vi "Periodic Tasks.vi"(8 "error in":errorcluster) -> ()   [LabVIEW 2012]
doc: "This VI runs in parallel to other tasks. It can contain as many user-defined periodic loops as you need. These can carry out PID or other sorts of timed response."
uses:
  <vilib>/Rock Robotics/SystemInterfaces/Utilities/FPGA_UtilitiesLED Source.ctl
  <vilib>/Rock Robotics/SystemInterfaces/Utilities/FPGA_UtilitiesLED State.ctl
  <vilib>/Rock Robotics/WPI/Compressor/WPI_CompressorGetSetRefNum.vi
  Robot Global Data.vi
panel:
  out "Shooter Speed":dbl
  out "Shooter Distance":dbl
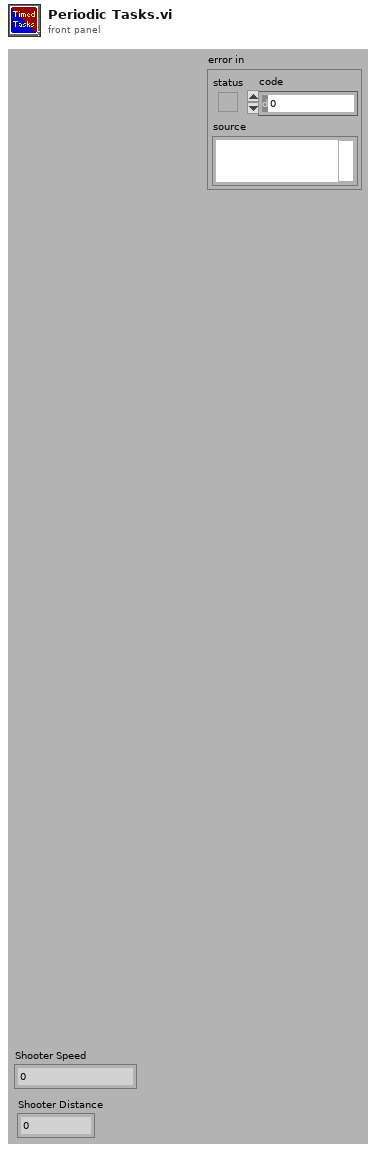
[diagram p1: front panel]
types:
  T1 = typedef "WPI_DriverStationRobotMode2.ctl" = enum16{"Autonomous Disabled", "Autonomous Enabled", "Teleop Disabled", "Teleop Enabled", "Timeout", "Finish", "Test Disabled", "Test Enabled"}
  T2 = typedef "WPI_EncoderDevRef.ctl" = cluster{"DevStatus":errorcluster, "EncoderIndex":T3, "CounterIndex":T4, "DistancePerCount":dbl, "Decoding Type":T5}
  T3 = typedef "FPGA_EncoderIdx.ctl" = enum8{"Enc 0", "Enc 1", "Enc 2", "Enc 3", "Invalid"}
  T4 = typedef "FPGA_CounterCtrSystemIndex.ctl" = enum8{"Ctr 0", "Ctr 1", "Ctr 2", "Ctr 3", "Ctr 4", "Ctr 5", "Ctr 6", "Ctr 7", "Invalid"}
  T5 = typedef "WPI_EncoderType.ctl" = enum16{"1x", "2x", "4x"}
  T6 = enum16{"Off", "Close Pyramid 3pt", "Far Pyramid 3pt", "Feeder Shot"}
  T7 = typedef "WPI_GyroDevRef.ctl" = cluster{"DevStatus":errorcluster, "Analog Module":T8, "Analog Channel":T9, "Offset":dbl, "Gain (VoltsPerDegree/Second)":dbl}
  T8 = typedef "FPGA_TypedefAnalogModule.ctl" = enum16{"Analog Module 1", "Analog Module 2"}
  T9 = typedef "FPGA_AIChannel.ctl" = enum8{"AI 1", "AI 2", "AI 3", "AI 4", "AI 5", "AI 6", "AI 7", "AI 8", "Invalid"}
  T10 = typedef "FPGA_UtilitiesLED State.ctl" = enum16{"Off", "On", "Toggle"}
  T11 = typedef "FPGA_UtilitiesLED Source.ctl" = enum16{"User LED", "FPGA LED"}
  T12 = typedef "WPI_CompressorDevRef.ctl" = cluster{"DevStatus":errorcluster, "DigitalInputDevRef":T13, "RelayDevRef":T16}
  T13 = typedef "WPI_DigitalInputDevRef.ctl" = cluster{"DevStatus":errorcluster, "DIO Channel":T14, "Digital Module":T15}
  T14 = typedef "FPGA_DIOChannel.ctl" = enum8{"DIO 1", "DIO 2", "DIO 3", "DIO 4", "DIO 5", "DIO 6", "DIO 7", "DIO 8", "DIO 9", "DIO 10", "DIO 11", "DIO 12", "DIO 13", "DIO 14", "Invalid"}
  T15 = typedef "FPGA_TypedefDigitalModule.ctl" = enum16{"Digital Module 1", "Digital Module 2"}
  T16 = typedef "WPI_RelayDevRef.ctl" = cluster{"DevStatus":errorcluster, "Relay Channel":T17, "Digital Module":T15, "Relay Direction":T18}
  T17 = typedef "FPGA_DIORelayChannel.ctl" = enum8{"Relay 1", "Relay 2", "Relay 3", "Relay 4", "Relay 5", "Relay 6", "Relay 7", "Relay 8", "Invalid"}
  T18 = typedef "WPI_RelayDirection.ctl" = enum16{"Both directions", "Forward only", "Reverse only"}
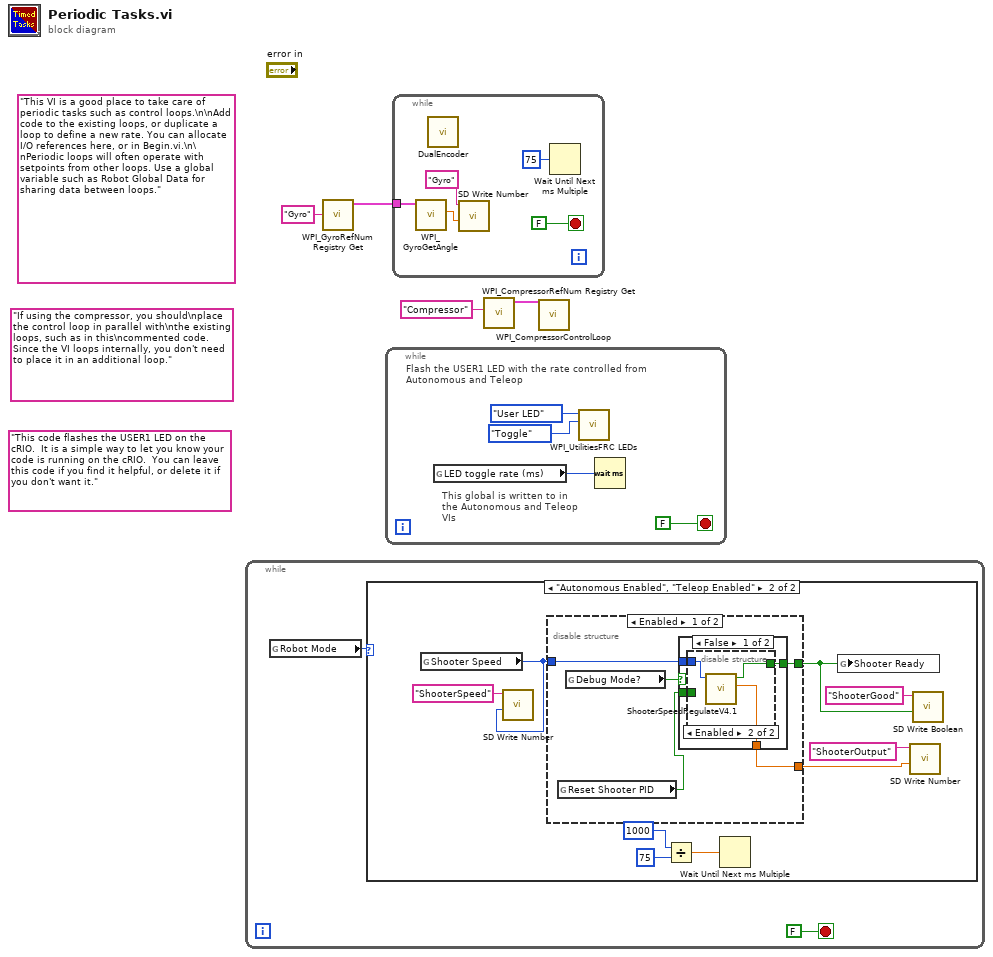
[diagram p0: block diagram]
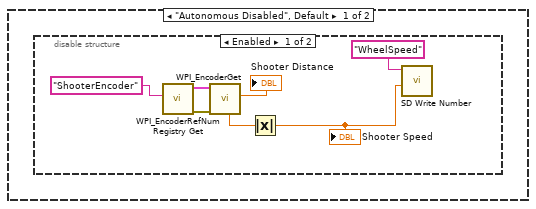
[diagram p2: hidden frame]
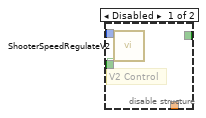
[diagram p4: hidden frame]
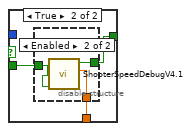
[diagram p5: hidden frame]
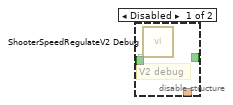
[diagram p6: hidden frame]
diagram:
  (unwired) "If using the compressor, you should\nplace the control loop in parallel with\nthe existing loops, such as in this\ncommented code. Since the VI loops internally, you don't need to place it in an additional loop."
  (unwired) "This code flashes the USER1 LED on the cRIO.  It is a simple way to let you know your code is running on the cRIO.  You can leave this code if you find it helpful, or delete it if you don't want it."
  (unwired) "This VI is a good place to take care of periodic tasks such as control loops.\n\nAdd code to the existing loops, or duplicate a loop to define a new rate. You can allocate I/O references here, or in Begin.vi.\n\nPeriodic loops will often operate with setpoints from other loops. Use a global variable such as Robot Global Data for sharing data between loops."
  n1 = while {
    stop <- FALSE stop-if-true
    n2 = global read "Robot Global Data.vi" "Robot Mode"() -> (w5:T1)
    n3 = case shown="\"Autonomous Enabled\", \"Teleop Enabled\"" w5 {
      frame "Autonomous Disabled", Default {
        n4 = disable-structure shown="Enabled" {
          frame Enabled {
            n5 = call <vilib>:"WPI_EncoderRefNum Registry Get.vi"("refnum name"="ShooterEncoder") -> ("error out"=w11:errorcluster, "EncoderDevRef"=w12:T2)  [unwired: 9 in]
            n6 = call <vilib>:"WPI_EncoderGet.vi"("error in (no error)"=w11, "EncoderDevRef"=w12) -> ("Distance"=→"Shooter Distance":dbl, "Rate"=w10:dbl)  [unwired: 4 in, 4 out]
            n7 = Absolute Value(x=w10) -> (abs(x)=w8:dbl)
            "Shooter Speed" <- w8
            n8 = call <vilib>:"SD Write Number.vi"("Numeric"=w8, "Name"="WheelSpeed") -> ()  [unwired: 8 in, 2 out]
          }
          frame Disabled {
          }
        }
      }
      frame "Autonomous Enabled", "Teleop Enabled" {
        n9 = global read "Robot Global Data.vi" "Shooter Speed"() -> (w18:T6)
        n10 = call <vilib>:"SD Write Number.vi"("Numeric"=w18, "Name"="ShooterSpeed") -> ()  [unwired: 8 in, 2 out]
        n11 = disable-structure shown="Enabled" {
          disable-tunnel: w18 -> [w27 _]
          disable-tunnel: [w24 _] -> w16
          disable-tunnel: [w23 _] -> w14
          frame Enabled {
            n12 = global read "Robot Global Data.vi" "Reset Shooter PID"() -> (w25:bool)
            n13 = global read "Robot Global Data.vi" "Debug Mode?"() -> (w26:bool)
            n14 = case shown="False" w26 {
              tunnel: w27 -> [w31 _]
              tunnel: w25 -> [w30 w39]
              tunnel: [w29 w38] -> w24
              tunnel: [w28 w37] -> w23
              frame False {
                n15 = disable-structure shown="Enabled" {
                  disable-tunnel: w31 -> [w33 w36]
                  disable-tunnel: w30 -> [w32 _]
                  disable-tunnel: [_ w35] -> w29
                  disable-tunnel: [_ w34] -> w28
                  frame Disabled {
                    # "V2 Control"
                    n16 = call "ShooterSpeedRegulateV2.vi"("Shooter Speed"=w33, "Reset Shooter PID"=w32) -> ()  [unwired: 12 in, 2 out]
                  }
                  frame Enabled {
                    n17 = call "ShooterSpeedRegulateV4.1.vi"("Shooter Speed"=w36) -> ("Voltage Output"=w34:dbl, "GO GO GO"=w35:bool)  [unwired: 9 in]
                  }
                }
              }
              frame True {
                n18 = disable-structure shown="Enabled" {
                  disable-tunnel: w39 -> [w40 w43]
                  disable-tunnel: [_ w42] -> w38
                  disable-tunnel: [_ w41] -> w37
                  frame Disabled {
                    # "V2 debug"
                    n19 = call "ShooterSpeedRegulateV2 Debug.vi"("Reset Shooter PID"=w40) -> ()  [unwired: 13 in, 2 out]
                  }
                  frame Enabled {
                    n20 = call "ShooterSpeedDebugV4.1.vi"("Reset PID"=w43) -> ("Wheel 1 Actual Voltage"=w41:dbl, "GO GO GO"=w42:bool)  [unwired: 9 in]
                  }
                }
              }
            }
          }
          frame Disabled {
          }
        }
        n21 = Divide(x=1000, y=75) -> (x/y=w20:dbl)
        n22 = Wait Until Next ms Multiple(millisecond multiple=w20) -> ()  [unwired: 1 out]
        n23 = global write "Robot Global Data.vi" "Shooter Ready"(w16) -> ()
        n24 = call <vilib>:"SD Write Number.vi"("Numeric"=w14, "Name"="ShooterOutput") -> ()  [unwired: 8 in, 2 out]
        n25 = call <vilib>:"SD Write Boolean.vi"("Boolean"=w16, "Name"="ShooterGood") -> ()  [unwired: 8 in, 2 out]
      }
    }
  }
  n26 = call <vilib>:"WPI_GyroRefNum Registry Get.vi"("refnum name"="Gyro") -> ("GyroDevRef"=w3:T7)  [unwired: 9 in, 1 out]
  n27 = while {
    stop <- FALSE stop-if-true
    # "This global is written to in the Autonomous and Teleop VIs"
    # "Flash the USER1 LED with the rate controlled from Autonomous and Teleop"
    n28 = global read "Robot Global Data.vi" "LED toggle rate (ms)"() -> (w44:u32)
    n29 = call <vilib>:"WPI_UtilitiesFRC LEDs.vi"("State"=FPGA_UtilitiesLED_State."Toggle", "LED Type"=FPGA_UtilitiesLED_Source."User LED") -> ()  [unwired: 1 in, 9 out]
    n30 = Wait (ms)(milliseconds to wait=w44) -> ()  [unwired: 1 out]
  }
  n31 = while {
    tunnel: w3 -> [w50]
    stop <- FALSE stop-if-true
    n32 = call <vilib>:"WPI_GyroGetAngle.vi"("GyroDevRef"=w50) -> ("Angle"=w49:dbl)  [unwired: 7 in, 3 out]
    n33 = call "DualEncoder.vi"() -> ()  [unwired: 8 in, 4 out]
    n34 = call <vilib>:"SD Write Number.vi"("Numeric"=w49, "Name"="Gyro") -> ()  [unwired: 8 in, 2 out]
    n35 = Wait Until Next ms Multiple(millisecond multiple=u32 75 ("milliseconds to wait")) -> ()  [unwired: 1 out]
  }
  n36 = call <vilib>:"WPI_CompressorRefNum Registry Get.vi"("refnum name"="Compressor") -> ("CompressorDevRef"=w2:T12)  [unwired: 9 in, 1 out]
  n37 = call <vilib>:"WPI_CompressorControlLoop.vi"("CompressorDevRef"=w2) -> ()  [unwired: 11 in]
